vi "fpga_W&R_oneADC_W_one_DAC.vi"() -> ()   [LabVIEW 2018]
uses:
  <vilib>/rvi/Emulation/niFpgaGetClockAttributes.vi
  <vilib>/rvi/Emulation/niFpgaSctlEmulationGetInTimedLoop.vi
  <vilib>/rvi/Emulation/niFpgaEmulationReportErrorSimple.vi
  <vilib>/rvi/eio/common/nirviEmuTemplateMethod_errors.vi
  <vilib>/rvi/Emulation/niFpgaCriticalErrorInLSC.vi
  <vilib>/eio/EIONode/EIONode.xnode
panel:
  in  "DAC 1 write":bool[](array[boolean])=[FALSE, FALSE, FALSE, FALSE, FALSE, FALSE, FALSE, FALSE, FALSE, FALSE, FALSE, FALSE, FALSE, FALSE, FALSE, FALSE]
  out "ADC CH1 read":bool[](array[boolean])
  in  "ADC CH1 write":bool[](array[boolean])=[FALSE, FALSE, FALSE, FALSE, FALSE, FALSE, FALSE, FALSE, FALSE, FALSE, FALSE, FALSE, FALSE, FALSE, FALSE, FALSE]
  in  "delay (us)":u32=40000
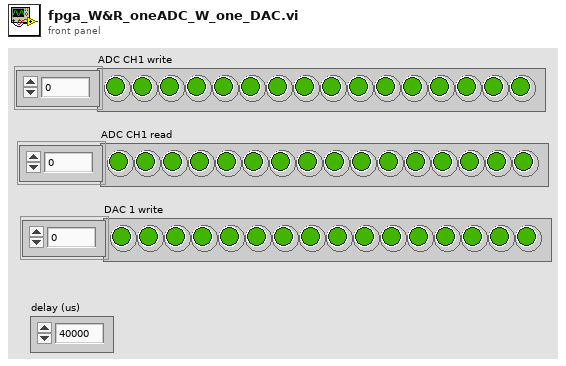
[diagram p1: front panel]
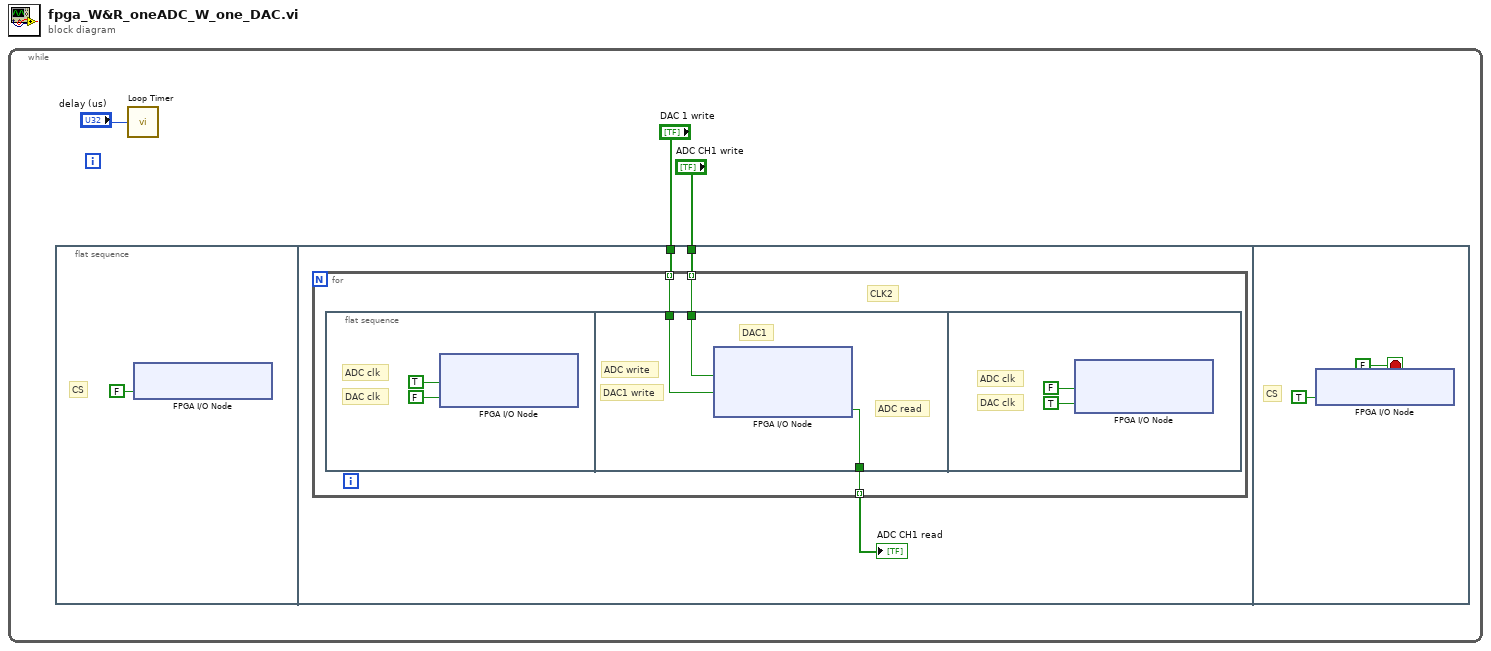
[diagram p0: block diagram]
diagram:
  n1 = while {
    stop <- FALSE stop-if-true
    n2 = flat-sequence {
      tunnel: "DAC 1 write" -> [w8]
      tunnel: "ADC CH1 write" -> [w7]
      frame #0 {
        # "CS"
        n3 = xnode "FPGA I/O Node"("ConnectorA/DIO4"=FALSE) -> ()  [unwired: 1 in, 1 out]
      }
      frame #1 {
        n4 = for {
          tunnel: w8 -> [w11] mode=indexing
          tunnel: w7 -> [w10] mode=indexing
          tunnel: [w9] -> w6 mode=indexing
          # "CLK2"
          n5 = flat-sequence {
            tunnel: w11 -> [w16]
            tunnel: w10 -> [w15]
            tunnel: [w14] -> w9
            frame #0 {
              # "DAC clk"
              # "ADC clk"
              n6 = xnode "FPGA I/O Node"("ConnectorA/DIO3"=TRUE, "ConnectorA/DIO5"=FALSE) -> ()  [unwired: 2 in, 2 out]
            }
            frame #1 {
              # "ADC read"
              # "DAC1 write"
              # "ADC write"
              # "DAC1"
              n7 = xnode "FPGA I/O Node"("ConnectorA/DIO2"=w15, "ConnectorA/DIO6"=w16) -> ("ConnectorA/DIO1"=w14:bool)  [unwired: 3 in, 3 out]
            }
            frame #2 {
              # "DAC clk"
              # "ADC clk"
              n8 = xnode "FPGA I/O Node"("ConnectorA/DIO3"=FALSE, "ConnectorA/DIO5"=TRUE) -> ()  [unwired: 2 in, 2 out]
            }
          }
        }
        "ADC CH1 read" <- w6
      }
      frame #2 {
        # "CS"
        n9 = xnode "FPGA I/O Node"("ConnectorA/DIO4"=TRUE) -> ()  [unwired: 1 in, 1 out]
      }
    }
    n10 = call "Loop Timer"("Count(Ticks)"="delay (us)") -> ()  [unwired: 1 out]
  }
